vi "YokoGS200 Get FuncAndRg.vi"(8 "error in (no error)":errorcluster, 11 "VISA Rsrc":refnum<visa-resource-name>="SR530") -> (0 "error out":errorcluster, 1 "Source Range":T1(ring), 2 "Source Function":enum16{"Current", "Voltage"}(ring), 3 "VISA Rsrc Out":refnum<visa-resource-name>="GPIB0::12::INSTR", 4 "ChaineRep":string caption="Chaîne de réponse")   [LabVIEW 2019]
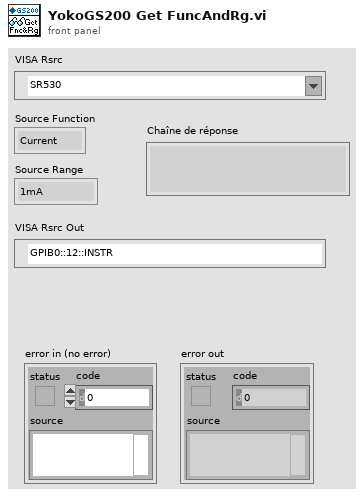
[diagram p1: front panel]
types:
  T1 = enum16{"1mA", "10mA", "100mA", "200mA", "10mV", "100mV", "1V", "10V", "30V", "Minimum", "Maximum"}
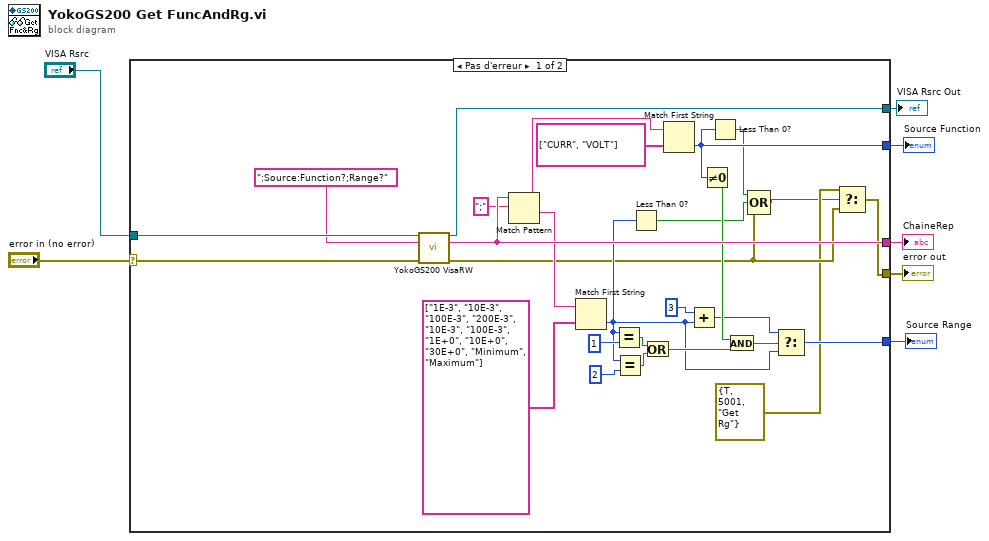
[diagram p0: block diagram]
diagram:
  n1 = case shown="Pas d'erreur" "error in (no error)" {
    selector: "error in (no error)" -> [w34 w36]
    tunnel: "VISA Rsrc" -> [w35 w37]
    tunnel: [w11 w36] -> w5
    tunnel: [w33 w37] -> w4
    tunnel: [w31 _] -> w3
    tunnel: [w14 _] -> w2
    tunnel: [w16 _] -> w1
    frame No Error {
      n2 = call <userlib>:"YokoGS200 VisaRW.vi"("VISA Rsrc"=w35, "ChaineCom"=":Source:Function?;Range?", "error in (no error)"=w34) -> ("VISA Rsrc Out"=w33:refnum<visa-resource-name>, "ChaineRep"=w31:string, "error out"=w10:errorcluster)  [unwired: 8 in, 2 out]
      n3 = Match Pattern(string=w31, regular expression=";") -> (before substring=w29:string, after substring=w26:string)  [unwired: 1 in, 2 out]
      n4 = Match First String(2:string[] ["1E-3", "10E-3", "100E-3", "200E-3", "10E-3", "100E-3", "1E+0", "10E+0", "30E+0", "Minimum", "Maximum"] ("output array"), 3:w26) -> (0:w15:i32)  [unwired: 1 out]
      n5 = Equal?(x=w15, y=1 ("index")) -> (x = y?=w23:bool)
      n6 = Equal?(x=w15, y=2 ("index")) -> (x = y?=w22:bool)
      n7 = Less Than 0?(x=w15) -> (x < 0?=w13:bool)
      n8 = Or(x=w23, y=w22) -> (x .or. y?=w21:bool)
      n9 = Match First String(2:string[] ["CURR", "VOLT"] ("string array"), 3:w29) -> (0:w14:i32)  [unwired: 1 out]
      n10 = Add(x=3, y=w15) -> (x+y=w18:i32)
      n11 = Not Equal To 0?(x=w14) -> (x != 0?=w20:bool)
      n12 = Less Than 0?(x=w14) -> (x < 0?=w12:bool)
      n13 = And(x=w20, y=w21) -> (x .and. y?=w19:bool)
      n14 = Compound Arithmetic op=OR(w12, w13, w10) -> (w8:bool)
      n15 = Select(t=w18, s=w19, f=w15) -> (s? t:f=w16:i32)
      n16 = Select(t=errorcluster {"status"=TRUE, "code"=5001, "source"="Get Rg"} ("error out"), s=w8, f=w10) -> (s? t:f=w11:errorcluster)
    }
    frame Error {
    }
  }
  "error out" <- w5
  "VISA Rsrc Out" <- w4
  "ChaineRep" <- w3
  "Source Function" <- w2
  "Source Range" <- w1
